vi "Status Current Temperature.vi"(8 "error in (no error)":errorcluster, 11 "heater_parent in":refnum<class "heater_parent.lvclass">) -> (0 "error out":errorcluster, 2 "Current Temperature":dbl, 3 "heater_parent out":refnum<class "heater_parent.lvclass">)   [LabVIEW 2020, in "polar_bear_plus_drivers.lvlib" / "heater_parent.lvclass"]
doc: "Get the current temperature reading."
uses:
  <instrlib>/RxnRover/Driver Polar Bear Plus/heater_parent/heater_parent.lvclass
  <instrlib>/RxnRover/Driver Polar Bear Plus/heater_parent/heater_parent.lvclass/heater_parent.ctl
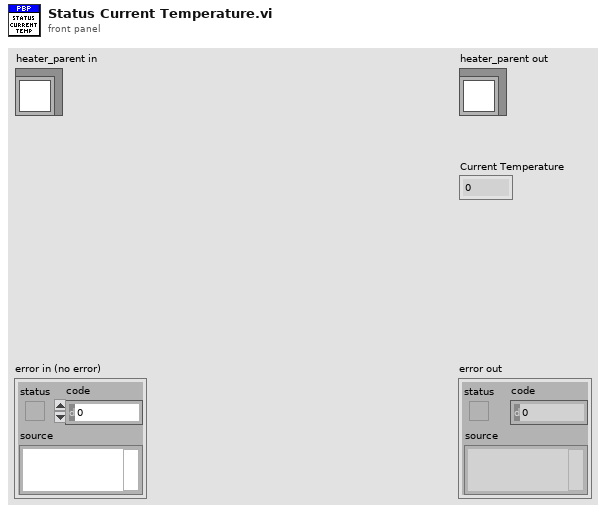
[diagram p1: front panel]
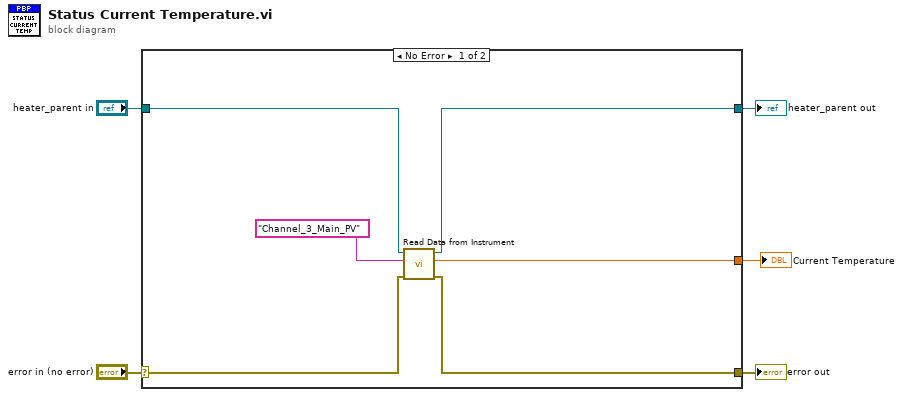
[diagram p0: block diagram]
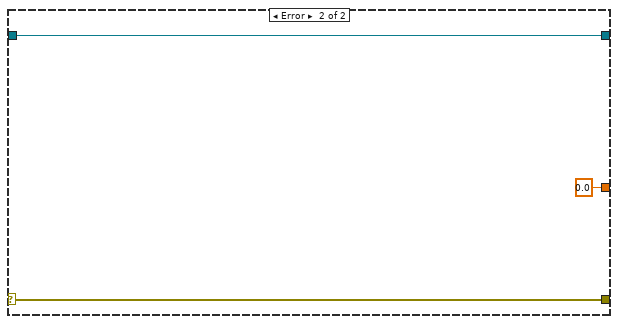
[diagram p2: hidden frame]
diagram:
  n1 = case shown="No Error" "error in (no error)" {
    selector: "error in (no error)" -> [w10 w14]
    tunnel: [w9 w14] -> w4
    tunnel: [w8 w13] -> w2
    tunnel: "heater_parent in" -> [w11 w13]
    tunnel: [w6 0.0 ("Value Read")] -> w1
    frame No Error {
      n2 = call-dynamic "Read Data from Instrument.vi"("error in (no error)"=w10, "Address"="Channel_3_Main_PV", "heater_parent in"=w11) -> ("error out"=w9:errorcluster, "Value Read"=w6:dbl, "heater_parent out"=w8:refnum<class "heater_parent.lvclass">)  [unwired: 6 in]
    }
    frame Error {
    }
  }
  "error out" <- w4
  "heater_parent out" <- w2
  "Current Temperature" <- w1
